vi "Autonomous Independent.vi"() -> ()   [LabVIEW 2016]
doc: "This VI is called when autonomous begins, and will automatically be terminated when autonomous ends. You can carry out timed or sensor driven robot movement independently without needing to return to the caller."
uses:
  <vilib>/Rock Robotics/WPI/Utilities/WPI_GetSetVariantRefNum.vi
  <vilib>/Rock Robotics/Network Tables/NT Read String.vi
  <vilib>/Rock Robotics/WPI/RobotDrive/WPI_RobotDriveArcadeDrive_Standard(NoSaturation).vi
  <vilib>/Rock Robotics/Network Tables/NT Write Numeric Array.vi
  <vilib>/Rock Robotics/Network Tables/NT Read Number.vi
  <vilib>/Rock Robotics/WPI/Ultrasonic/WPI_SonarMB1010AnalogRefNum Registry Get.vi
  <vilib>/Rock Robotics/WPI/Ultrasonic/WPI_SonarMB1010AnalogGetRange.vi
panel:
  out "Angle":dbl
  in  "Dial":dbl(knob) scale=-180.0..180.0
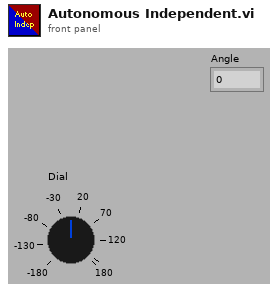
[diagram p1: front panel]
types:
  T1 = typedef "WPI_JoystickDevRef.ctl" = cluster{"Device":T2}
  T2 = typedef "WPI_JoystickDeviceEnum.ctl" = enum16{"USB 0", "USB 1", "USB 2", "USB 3", "USB 4", "USB 5"}
  T3 = typedef "WPI_RobotDriveDevRef.ctl" = cluster{"DevStatus":errorcluster, "Motors[]":T4[], "Square Inputs":bool, "Max Output":dbl}
  T4 = typedef "WPI_MotorControlDeviceRef.ctl" = cluster{"DeviceStatus":errorcluster, "Type":T5, "PWM":cluster{"PWM Channel":T6, "DeadBand":T7}, "CAN":cluster{"Device Number":u8, "SetOutput VI Ref":variant, "GetOutput VI Ref":variant, "Enable VI Ref":variant, "Disable VI Ref":variant, "Data":variant}, "Invert":bool}
  T5 = typedef "WPI_MotorControlType.ctl" = enum16{"PWM", "CAN"}
  T6 = typedef "FPGA_DIOPWMChannel.ctl" = enum8{"PWM 0", "PWM 1", "PWM 2", "PWM 3", "PWM 4", "PWM 5", "PWM 6", "PWM 7", "PWM 8", "PWM 9", "PWM MXP 0", "PWM MXP 1", "PWM MXP 2", "PWM MXP 3", "PWM MXP 4", "PWM MXP 5", "PWM MXP 6", "PWM MXP 7", "PWM MXP 8", "PWM MXP 9", "Invalid"}
  T7 = typedef "WPI_PWMDeadband.ctl" = cluster{"Name":string, "maxPositivePwm":i32, "minPositivePwm":i32, "centerPwm":i32, "maxNegativePwm":i32, "minNegativePwm":i32, "angularRange":u16}
  T8 = typedef "WPI_SonarMB1010AnalogDeviceRef.ctl" = cluster{"AIDeviceRef":T9, "Scaling factor (V/in)":dbl, "Average Bits":u8}
  T9 = typedef "WPI_AnalogChannelDevRef.ctl" = cluster{"DevStatus":errorcluster, "Analog Channel":T10}
  T10 = typedef "FPGA_AIChannel.ctl" = enum8{"AI 0", "AI 1", "AI 2", "AI 3", "AI MXP 0", "AI MXP 1", "AI MXP 2", "AI MXP 3", "Invalid"}
  T11 = typedef "WPI_GyroDevRef.ctl" = cluster{"DevStatus":errorcluster, "Analog Channel":T10, "Offset":dbl, "Gain (VoltsPerDegree/Second)":dbl, "Gyro Type":enum16{"Analog", "XRS450"}, "Handle":i32, "SPI Bus":T12, "Device Found":bool, "Sample Rate":dbl, "Calibrate On Open":bool}
  T12 = typedef "spi_bus.ctl" = enum16{"SPI On-Board, CS0", "SPI On-Board, CS1", "SPI On-Board, CS2", "SPI On-Board, CS3", "SPI MXP", "Invalid"}
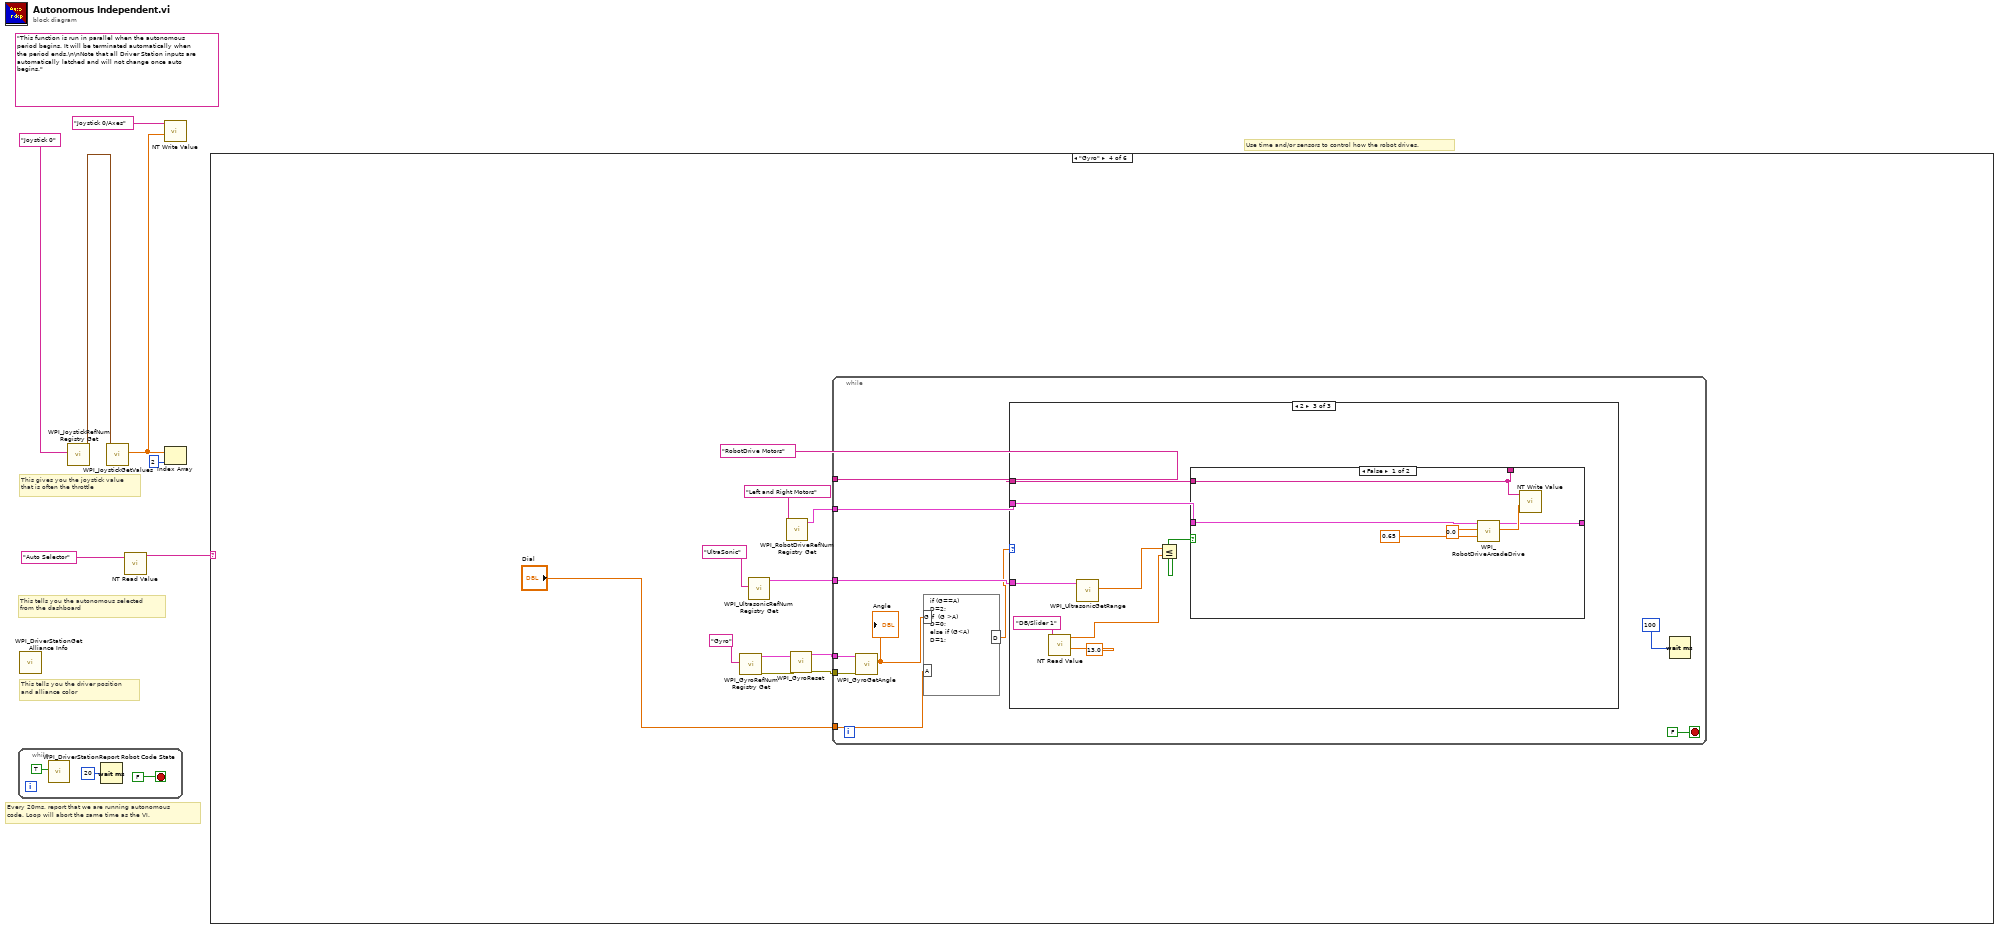
[diagram p0: block diagram]
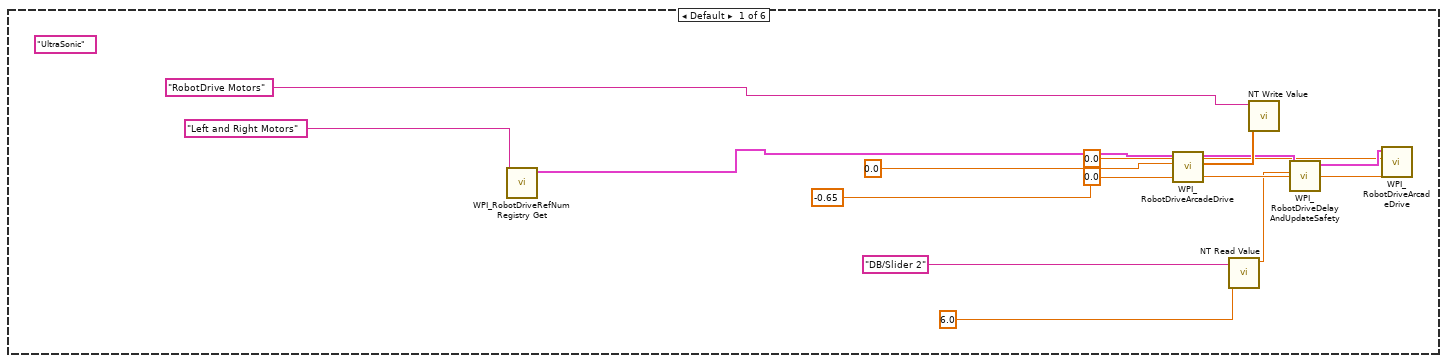
[diagram p2: hidden frame]
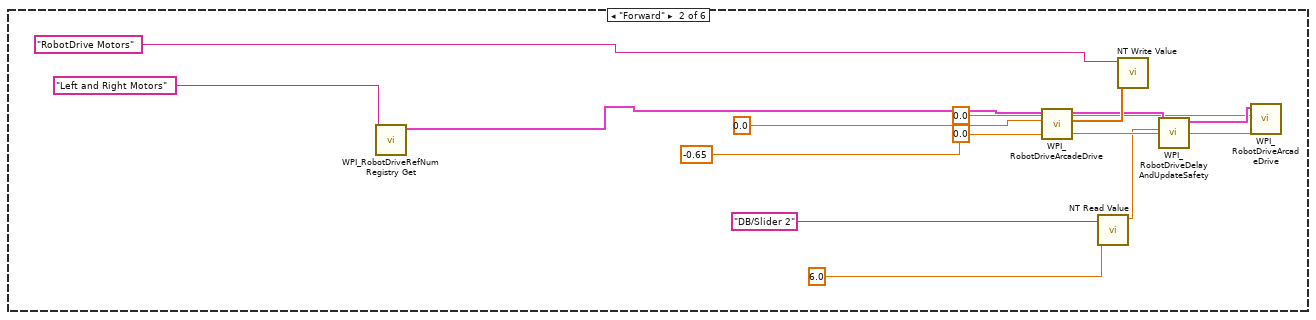
[diagram p3: hidden frame]
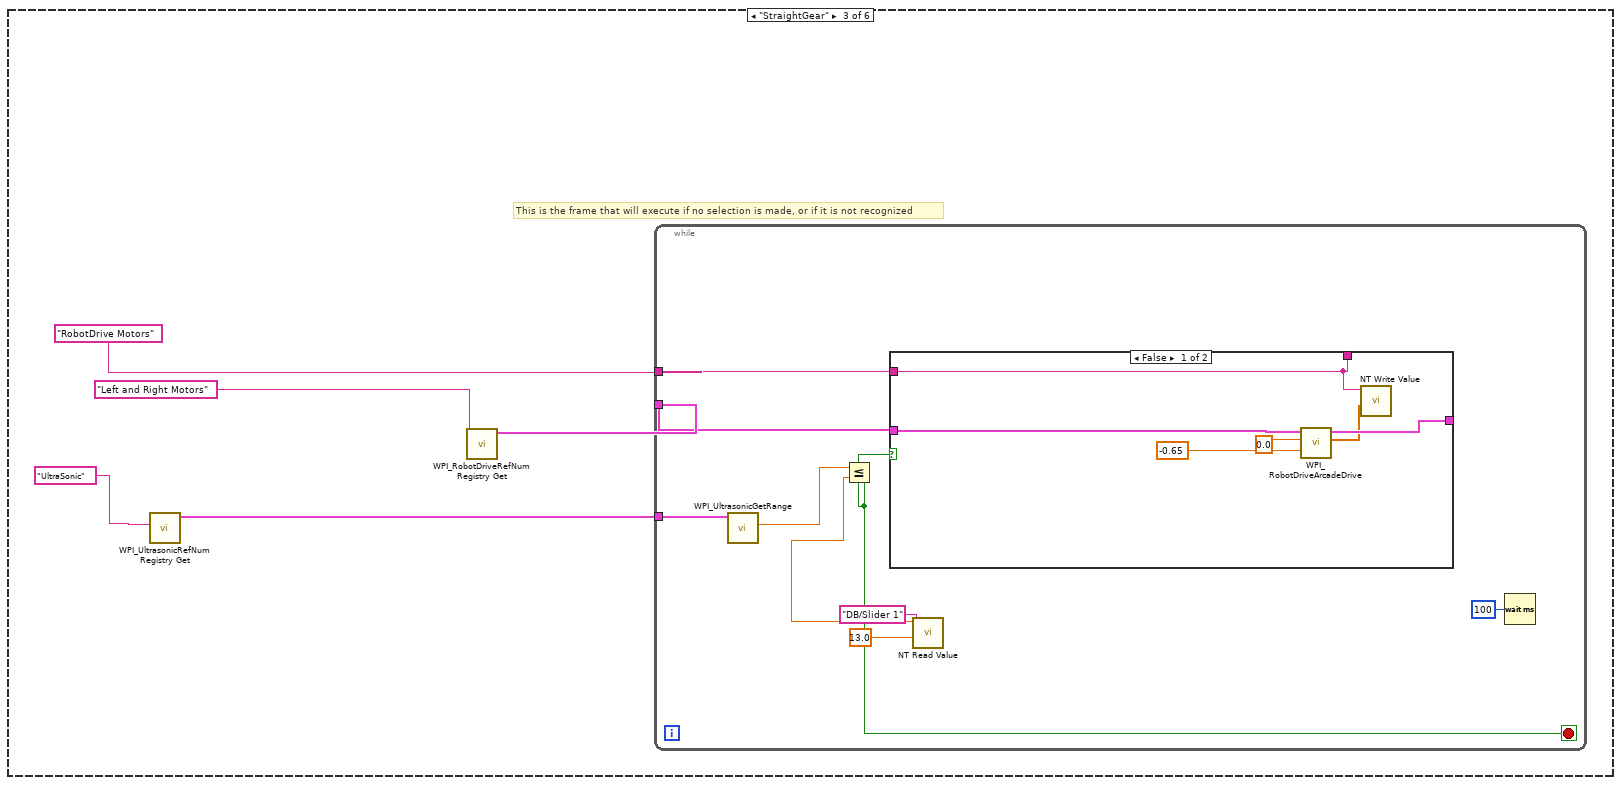
[diagram p4: hidden frame]
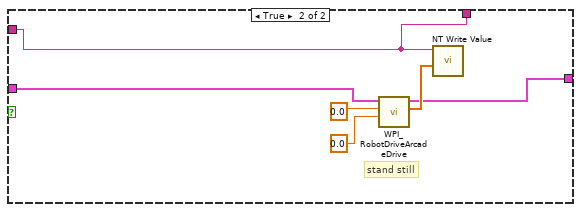
[diagram p5: hidden frame]
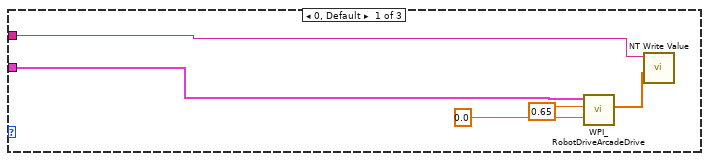
[diagram p6: hidden frame]
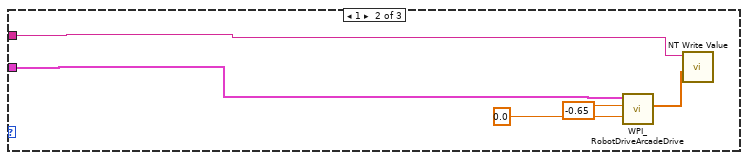
[diagram p7: hidden frame]
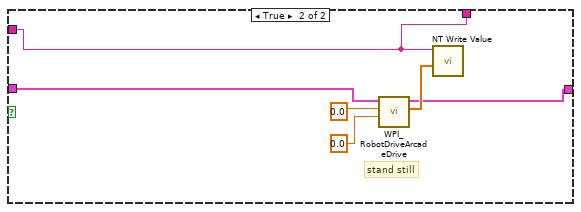
[diagram p8: hidden frame]
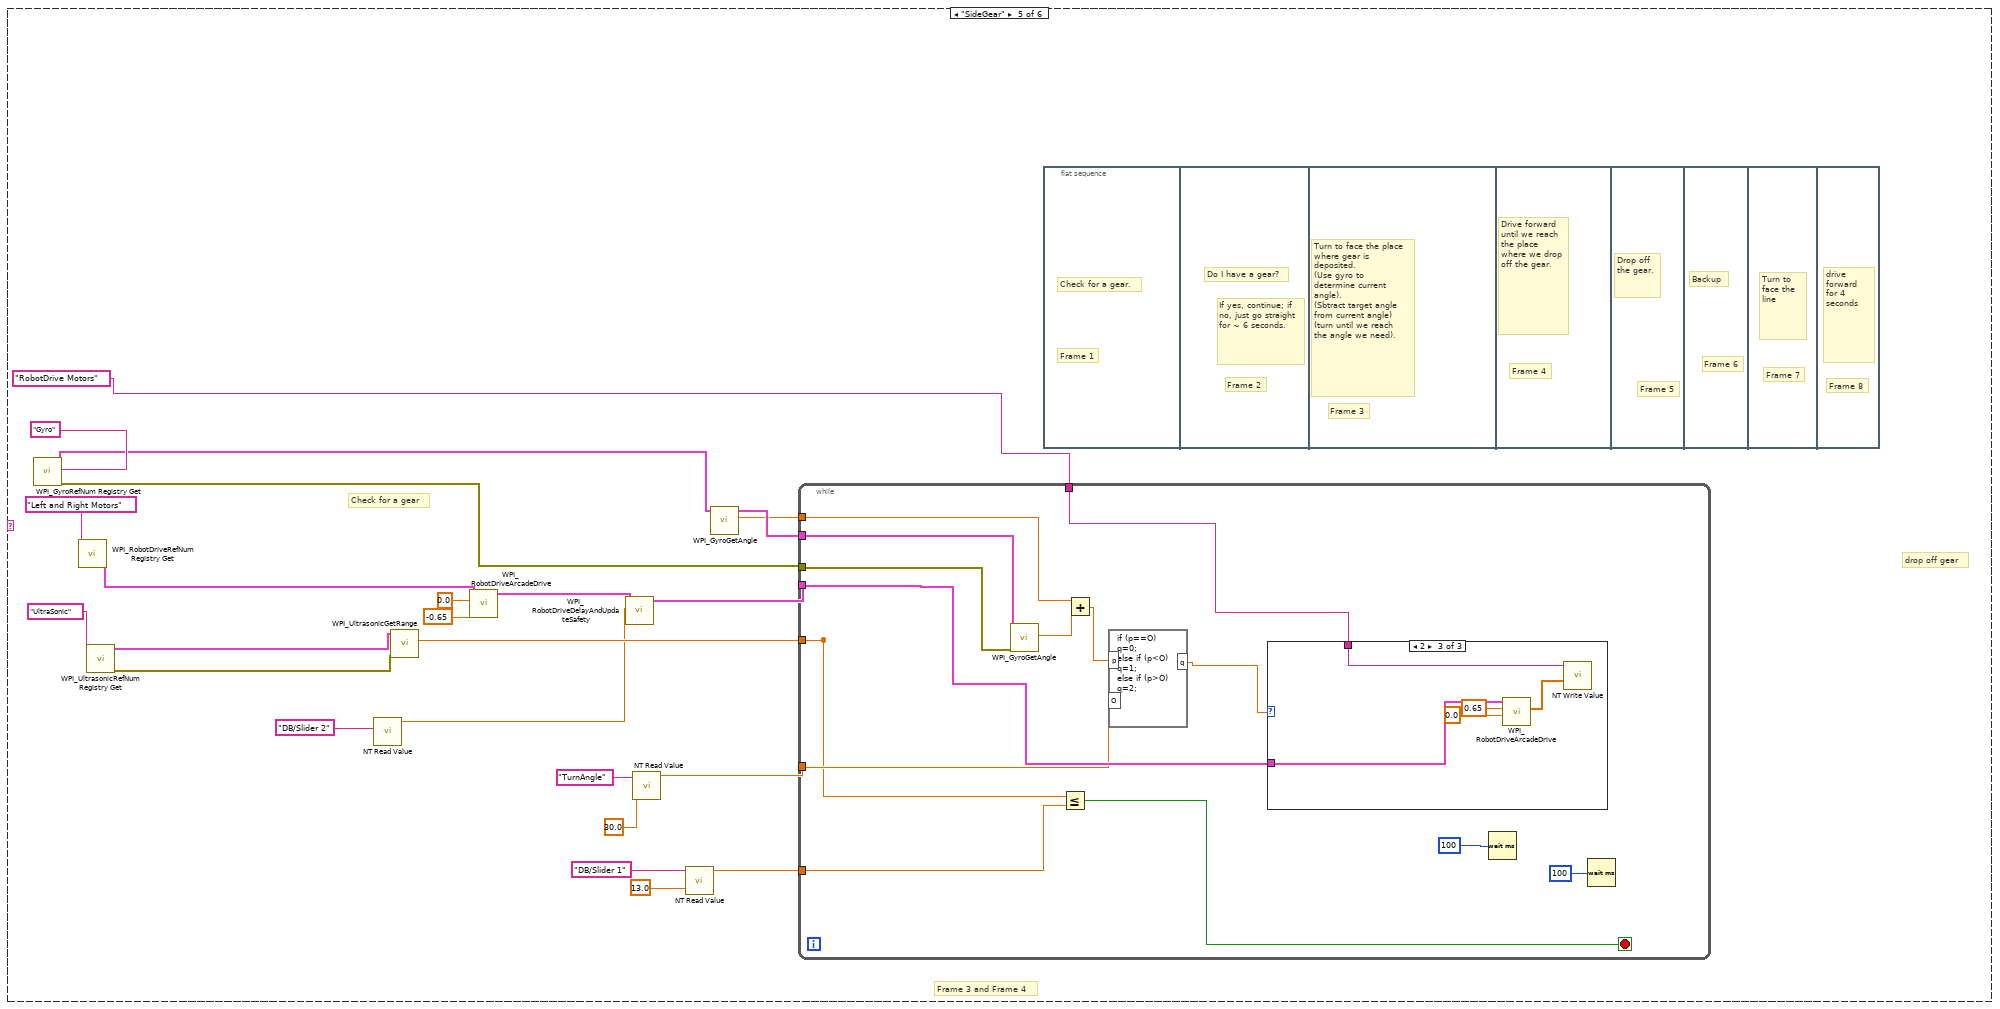
[diagram p9: hidden frame]
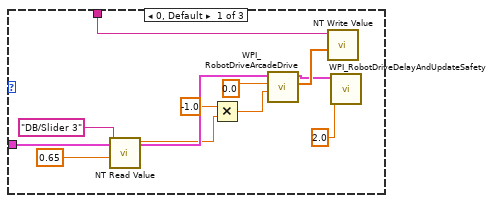
[diagram p10: hidden frame]
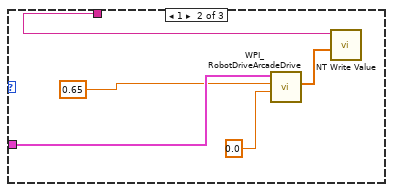
[diagram p11: hidden frame]
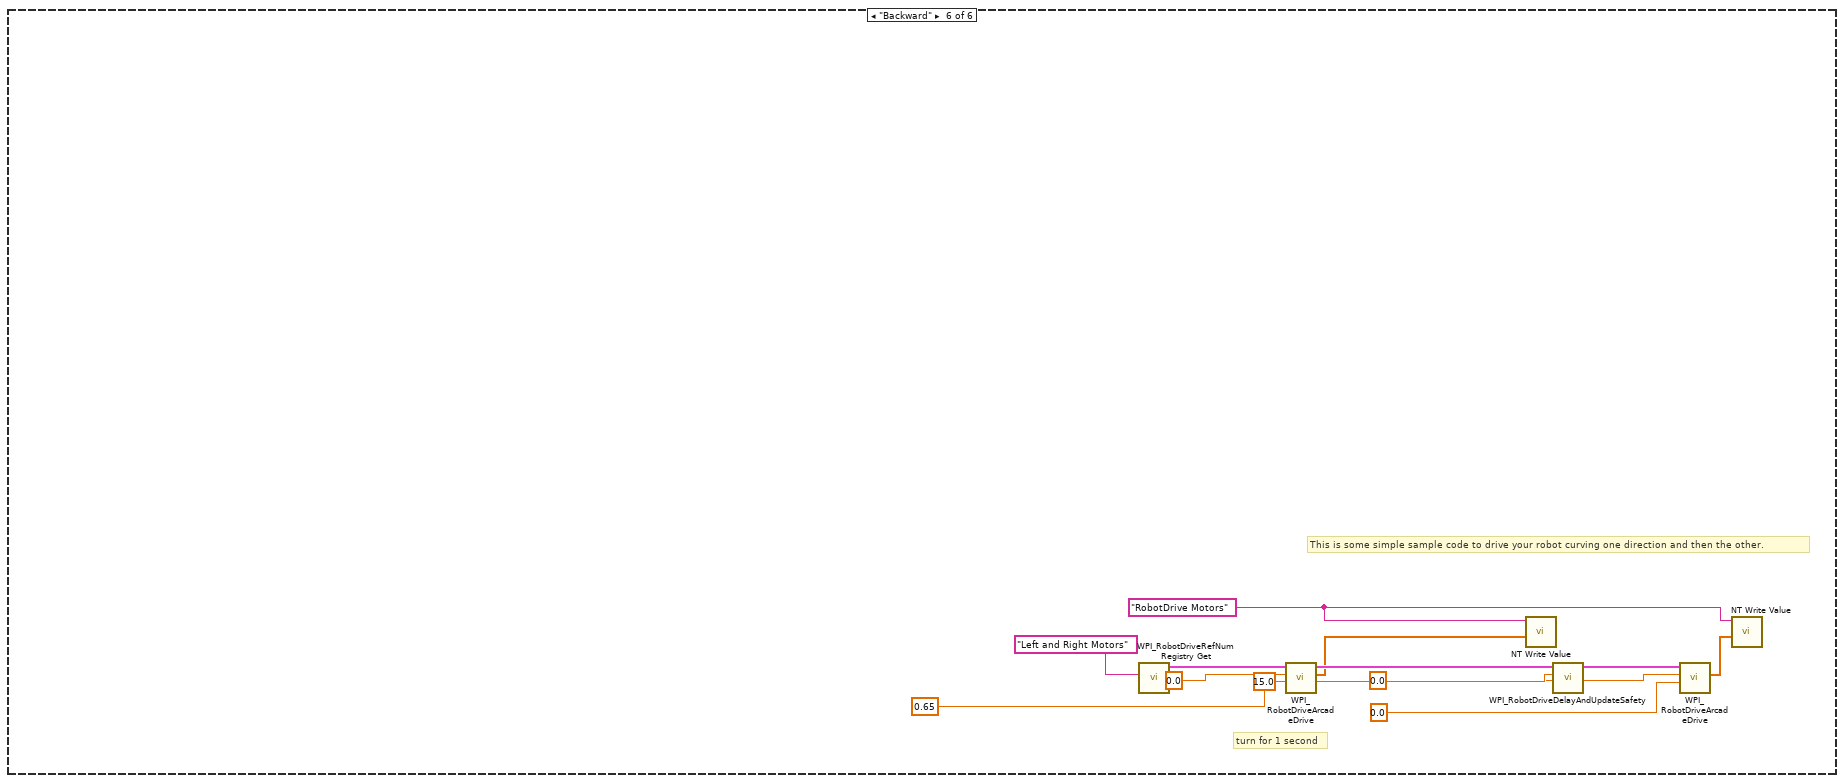
[diagram p12: hidden frame]
diagram:
  (unwired) "This function is run in parallel when the autonomous period begins. It will be terminated automatically when the period ends.\n\nNote that all Driver Station inputs are automatically latched and will not change once auto begins."
  # "This tells you the autonomous selected\nfrom the dashboard"
  # "Every 20ms, report that we are running autonomous\ncode. Loop will abort the same time as the VI."
  # "This gives you the joystick value\nthat is often the throttle"
  # "Use time and/or sensors to control how the robot drives."
  # "This tells you the driver position\nand alliance color"
  n1 = while {
    stop <- FALSE stop-if-true
    n2 = call <vilib>:"WPI_DriverStationReport Robot Code State.vi"("Autonomous"=TRUE) -> ()  [unwired: 10 in, 1 out]
    n3 = Wait (ms)(milliseconds to wait=u32 20) -> ()  [unwired: 1 out]
  }
  n4 = call <vilib>:"WPI_DriverStationGet Alliance Info.vi"() -> ()  [unwired: 12 out]
  n5 = call <vilib>:"WPI_JoystickRefNum Registry Get.vi"("refnum name"="Joystick 0") -> ("JoystickDevRef"=w6:T1)  [unwired: 1 in, 9 out]
  n6 = call <vilib>:"WPI_JoystickGetValues.vi"("JoystickDevRef"=w6) -> ("Axes"=w2:dbl[])  [unwired: 6 in, 4 out]
  n7 = call-poly <vilib>:"NT Read Value.vi"("Name"="Auto Selector") -> ("String"=w3:string)  [unwired: 9 in, 1 out]
  n8 = call-poly <vilib>:"NT Write Value.vi"("Numeric Array"=w2, "Name"="Joystick 0/Axes") -> ()  [unwired: 9 in, 1 out]
  n9 = Index Array(array=w2, index=2) -> ()  [unwired: 1 out]
  n10 = case shown="\"Gyro\"" w3 {
    frame Default {
      (unwired) "UltraSonic" ("refnum name")
      n11 = call <vilib>:"WPI_RobotDriveRefNum Registry Get.vi"("refnum name"="Left and Right Motors") -> ("RobotDriveDevRef"=w19:T3)  [unwired: 1 in, 9 out]
      n12 = call-poly <vilib>:"WPI_RobotDriveArcadeDrive.vi"("Y axis value"=-0.65, "X axis value"=0.0, "RobotDriveDevRef"=w19) -> ("Motor Values"=w20:dbl[], "RobotDriveDevRef"=w17:T3)  [unwired: 1 in, 6 out]
      n13 = call-poly <vilib>:"NT Read Value.vi"("Default Value"=6.0, "Name"="DB/Slider 2") -> ("Numeric"=w13:dbl)  [unwired: 8 in, 1 out]
      n14 = call-poly <vilib>:"NT Write Value.vi"("Numeric Array"=w20, "Name"="RobotDrive Motors") -> ()  [unwired: 9 in, 1 out]
      n15 = call <vilib>:"WPI_RobotDriveDelayAndUpdateSafety.vi"("Delay (s)"=w13, "RobotDriveDevRef"=w17) -> ("RobotDriveDevRef 2"=w16:T3)  [unwired: 8 in, 1 out]
      n16 = call-poly <vilib>:"WPI_RobotDriveArcadeDrive.vi"("Y axis value"=0.0, "X axis value"=0.0, "RobotDriveDevRef"=w16) -> ()  [unwired: 1 in, 8 out]
    }
    frame "Forward" {
      n17 = call <vilib>:"WPI_RobotDriveRefNum Registry Get.vi"("refnum name"="Left and Right Motors") -> ("RobotDriveDevRef"=w32:T3)  [unwired: 1 in, 9 out]
      n18 = call-poly <vilib>:"WPI_RobotDriveArcadeDrive.vi"("Y axis value"=-0.65, "X axis value"=0.0, "RobotDriveDevRef"=w32) -> ("Motor Values"=w33:dbl[], "RobotDriveDevRef"=w30:T3)  [unwired: 1 in, 6 out]
      n19 = call-poly <vilib>:"NT Read Value.vi"("Default Value"=6.0, "Name"="DB/Slider 2") -> ("Numeric"=w26:dbl)  [unwired: 8 in, 1 out]
      n20 = call-poly <vilib>:"NT Write Value.vi"("Numeric Array"=w33, "Name"="RobotDrive Motors") -> ()  [unwired: 9 in, 1 out]
      n21 = call <vilib>:"WPI_RobotDriveDelayAndUpdateSafety.vi"("Delay (s)"=w26, "RobotDriveDevRef"=w30) -> ("RobotDriveDevRef 2"=w29:T3)  [unwired: 8 in, 1 out]
      n22 = call-poly <vilib>:"WPI_RobotDriveArcadeDrive.vi"("Y axis value"=0.0, "X axis value"=0.0, "RobotDriveDevRef"=w29) -> ()  [unwired: 1 in, 8 out]
    }
    frame "StraightGear" {
      # "This is the frame that will execute if no selection is made, or if it is not recognized"
      n23 = call-poly <vilib>:"WPI_UltrasonicRefNum Registry Get.vi"("refnum name"="UltraSonic") -> ("SonarMB1010AnalogDevRef"=w38:T8)  [unwired: 9 in, 1 out]
      n24 = call <vilib>:"WPI_RobotDriveRefNum Registry Get.vi"("refnum name"="Left and Right Motors") -> ("RobotDriveDevRef"=w39:T3)  [unwired: 1 in, 9 out]
      n25 = while {
        tunnel: "RobotDrive Motors" ("Name") -> [w50]
        tunnel: w39 -> [w49]
        tunnel: w38 -> [w47]
        stop <- w42 stop-if-true
        n26 = call-poly <vilib>:"WPI_UltrasonicGetRange.vi"("SonarMB1010AnalogDevRef"=w47) -> ("Distance"=w48:dbl)  [unwired: 8 in, 2 out]
        n27 = call-poly <vilib>:"NT Read Value.vi"("Default Value"=13.0, "Name"="DB/Slider 1") -> ("Numeric"=w43:dbl)  [unwired: 8 in, 1 out]
        n28 = Less Or Equal?(x=w48, y=w43) -> (x <= y?=w42:bool)
        n29 = case shown="False" w42 {
          tunnel: w50 -> [w55 w57]
          tunnel: [w55 w57] -> _
          tunnel: w49 -> [w54 w59]
          tunnel: [w53 w58] -> _
          frame False {
            n30 = call-poly <vilib>:"WPI_RobotDriveArcadeDrive.vi"("Y axis value"=-0.65, "X axis value"=0.0, "RobotDriveDevRef"=w54) -> ("Motor Values"=w51:dbl[], "RobotDriveDevRef"=w53:T3)  [unwired: 1 in, 6 out]
            n31 = call-poly <vilib>:"NT Write Value.vi"("Numeric Array"=w51, "Name"=w55) -> ()  [unwired: 9 in, 1 out]
          }
          frame True {
            # "stand still"
            n32 = call-poly <vilib>:"WPI_RobotDriveArcadeDrive.vi"("Y axis value"=0.0 ("X axis value"), "X axis value"=0.0, "RobotDriveDevRef"=w59) -> ("Motor Values"=w62:dbl[], "RobotDriveDevRef"=w58:T3)  [unwired: 1 in, 6 out]
            n33 = call-poly <vilib>:"NT Write Value.vi"("Numeric Array"=w62, "Name"=w57) -> ()  [unwired: 9 in, 1 out]
          }
        }
        n34 = Wait (ms)(milliseconds to wait=u32 100) -> ()  [unwired: 1 out]
      }
    }
    frame "Gyro" {
      n35 = call <vilib>:"WPI_GyroRefNum Registry Get.vi"("refnum name"="Gyro") -> ("error out"=w66:errorcluster, "GyroDevRef"=w65:T11)  [unwired: 9 in]
      n36 = call-poly <vilib>:"WPI_UltrasonicRefNum Registry Get.vi"("refnum name"="UltraSonic") -> ("SonarMB1010AnalogDevRef"=w71:T8)  [unwired: 9 in, 1 out]
      n37 = call <vilib>:"WPI_RobotDriveRefNum Registry Get.vi"("refnum name"="Left and Right Motors") -> ("RobotDriveDevRef"=w68:T3)  [unwired: 1 in, 9 out]
      n38 = call <vilib>:"WPI_GyroReset.vi"("error in"=w66, "GyroDevRef"=w65) -> ("error out"=w67:errorcluster, "GyroDevRef"=w64:T11)  [unwired: 8 in]
      n39 = while {
        tunnel: "RobotDrive Motors" ("Name") -> [w83]
        tunnel: w68 -> [w79]
        tunnel: w71 -> [w77]
        tunnel: w64 -> [w81]
        tunnel: w67 -> [w80]
        tunnel: "Dial" -> [w75]
        stop <- FALSE stop-if-true
        n40 = call <vilib>:"WPI_GyroGetAngle.vi"("error in"=w80, "GyroDevRef"=w81) -> ("Angle"=w74:dbl)  [unwired: 5 in, 4 out]
        "Angle" <- w74
        n41 = formula code="if (G==A)\nD=2;\nif  (G >A)\nD=0;\nelse if (G<A)\nD=1;"("G"=w74, "A"=w75) -> ("D"=w76:dbl)
        n42 = case shown="2" w76 {
          tunnel: w83 -> [w84 w90 w100]
          tunnel: w79 -> [w85 w89 w99]
          tunnel: w77 -> [_ _ w97]
          frame 0, Default {
            n43 = call-poly <vilib>:"WPI_RobotDriveArcadeDrive.vi"("Y axis value"=0.0, "X axis value"=0.65, "RobotDriveDevRef"=w85) -> ("Motor Values"=w88:dbl[])  [unwired: 1 in, 7 out]
            n44 = call-poly <vilib>:"NT Write Value.vi"("Numeric Array"=w88, "Name"=w84) -> ()  [unwired: 9 in, 1 out]
          }
          frame 1 {
            n45 = call-poly <vilib>:"WPI_RobotDriveArcadeDrive.vi"("Y axis value"=0.0, "X axis value"=-0.65, "RobotDriveDevRef"=w89) -> ("Motor Values"=w91:dbl[])  [unwired: 1 in, 7 out]
            n46 = call-poly <vilib>:"NT Write Value.vi"("Numeric Array"=w91, "Name"=w90) -> ()  [unwired: 9 in, 1 out]
          }
          frame 2 {
            n47 = call-poly <vilib>:"NT Read Value.vi"("Default Value"=13.0, "Name"="DB/Slider 1") -> ("Numeric"=w94:dbl)  [unwired: 8 in, 1 out]
            n48 = call-poly <vilib>:"WPI_UltrasonicGetRange.vi"("SonarMB1010AnalogDevRef"=w97) -> ("Distance"=w98:dbl)  [unwired: 8 in, 2 out]
            n49 = Less Or Equal?(x=w98, y=w94) -> (x <= y?=w101:bool)
            n50 = case shown="False" w101 {
              tunnel: w100 -> [w106 w109]
              tunnel: [w106 w109] -> _
              tunnel: w99 -> [w105 w110]
              tunnel: [w102 w108] -> _
              frame False {
                n51 = call-poly <vilib>:"WPI_RobotDriveArcadeDrive.vi"("Y axis value"=0.65, "X axis value"=0.0, "RobotDriveDevRef"=w105) -> ("Motor Values"=w103:dbl[], "RobotDriveDevRef"=w102:T3)  [unwired: 1 in, 6 out]
                n52 = call-poly <vilib>:"NT Write Value.vi"("Numeric Array"=w103, "Name"=w106) -> ()  [unwired: 9 in, 1 out]
              }
              frame True {
                # "stand still"
                n53 = call-poly <vilib>:"WPI_RobotDriveArcadeDrive.vi"("Y axis value"=0.0 ("X axis value"), "X axis value"=0.0, "RobotDriveDevRef"=w110) -> ("Motor Values"=w113:dbl[], "RobotDriveDevRef"=w108:T3)  [unwired: 1 in, 6 out]
                n54 = call-poly <vilib>:"NT Write Value.vi"("Numeric Array"=w113, "Name"=w109) -> ()  [unwired: 9 in, 1 out]
              }
            }
          }
        }
        n55 = Wait (ms)(milliseconds to wait=u32 100) -> ()  [unwired: 1 out]
      }
    }
    frame "SideGear" {
      # "Check for a gear"
      # "Frame 3 and Frame 4"
      # "drop off gear"
      n56 = call <vilib>:"WPI_GyroRefNum Registry Get.vi"("refnum name"="Gyro") -> ("error out"=w132:errorcluster, "GyroDevRef"=w122:T11)  [unwired: 9 in]
      n57 = call <vilib>:"WPI_RobotDriveRefNum Registry Get.vi"("refnum name"="Left and Right Motors") -> ("RobotDriveDevRef"=w129:T3)  [unwired: 1 in, 9 out]
      n58 = call-poly <vilib>:"WPI_UltrasonicRefNum Registry Get.vi"("refnum name"="UltraSonic") -> ("error out"=w130:errorcluster, "SonarMB1010AnalogDevRef"=w134:T8)  [unwired: 9 in]
      n59 = call-poly <vilib>:"NT Read Value.vi"("Name"="DB/Slider 2") -> ("Numeric"=w124:dbl)  [unwired: 9 in, 1 out]
      n60 = call-poly <vilib>:"WPI_UltrasonicGetRange.vi"("error in"=w130, "SonarMB1010AnalogDevRef"=w134) -> ("Distance"=w133:dbl)  [unwired: 7 in, 2 out]
      n61 = call-poly <vilib>:"WPI_RobotDriveArcadeDrive.vi"("Y axis value"=-0.65, "X axis value"=0.0, "RobotDriveDevRef"=w129) -> ("RobotDriveDevRef"=w126:T3)  [unwired: 6 in, 2 out]
      n62 = call <vilib>:"WPI_RobotDriveDelayAndUpdateSafety.vi"("Delay (s)"=w124, "RobotDriveDevRef"=w126) -> ("RobotDriveDevRef 2"=w127:T3)  [unwired: 8 in, 1 out]
      n63 = call-poly <vilib>:"NT Read Value.vi"("Default Value"=30.0, "Name"="TurnAngle") -> ("Numeric"=w118:dbl)  [unwired: 8 in, 1 out]
      n64 = call-poly <vilib>:"NT Read Value.vi"("Default Value"=13.0, "Name"="DB/Slider 1") -> ("Numeric"=w116:dbl)  [unwired: 8 in, 1 out]
      n65 = call <vilib>:"WPI_GyroGetAngle.vi"("GyroDevRef"=w122) -> ("Angle"=w120:dbl, "GyroDevRef"=w121:T11)  [unwired: 6 in, 3 out]
      n66 = while {
        tunnel: w121 -> [w150]
        tunnel: w127 -> [w149]
        tunnel: "RobotDrive Motors" ("Name") -> [w145]
        tunnel: w132 -> [w148]
        tunnel: [w143] -> _
        tunnel: w118 -> [w144]
        tunnel: w133 -> [w143]
        tunnel: w120 -> [w142]
        tunnel: w116 -> [w139]
        stop <- w146 stop-if-true
        n67 = call <vilib>:"WPI_GyroGetAngle.vi"("error in"=w148, "GyroDevRef"=w150) -> ("Angle"=w141:dbl)  [unwired: 5 in, 4 out]
        n68 = Less Or Equal?(x=w143, y=w139) -> (x <= y?=w146:bool)
        n69 = Add(x=w142, y=w141) -> (x+y=w140:dbl)
        n70 = formula code="if (p==O)\nq=0;\nelse if (p<O)\nq=1;\nelse if (p>O)\nq=2;"("p"=w140, "O"=w144) -> ("q"=w147:dbl)
        n71 = case shown="2" w147 {
          tunnel: w149 -> [w158 w166 w171]
          tunnel: w145 -> [w157 w165 w168]
          frame 0, Default {
            n72 = call-poly <vilib>:"NT Read Value.vi"("Default Value"=0.65, "Name"="DB/Slider 3") -> ("Numeric"=w155:dbl)  [unwired: 8 in, 1 out]
            n73 = Multiply(x=-1.0, y=w155) -> (x*y=w156:dbl)
            n74 = call-poly <vilib>:"WPI_RobotDriveArcadeDrive.vi"("Y axis value"=w156, "X axis value"=0.0, "RobotDriveDevRef"=w158) -> ("Motor Values"=w160:dbl[], "RobotDriveDevRef"=w152:T3)  [unwired: 1 in, 6 out]
            n75 = call-poly <vilib>:"NT Write Value.vi"("Numeric Array"=w160, "Name"=w157) -> ()  [unwired: 9 in, 1 out]
            n76 = call <vilib>:"WPI_RobotDriveDelayAndUpdateSafety.vi"("Delay (s)"=2.0, "RobotDriveDevRef"=w152) -> ()  [unwired: 8 in, 2 out]
          }
          frame 1 {
            n77 = call-poly <vilib>:"WPI_RobotDriveArcadeDrive.vi"("Y axis value"=0.0, "X axis value"=0.65 ("Default Value"), "RobotDriveDevRef"=w166) -> ("Motor Values"=w167:dbl[])  [unwired: 1 in, 7 out]
            n78 = call-poly <vilib>:"NT Write Value.vi"("Numeric Array"=w167, "Name"=w165) -> ()  [unwired: 9 in, 1 out]
          }
          frame 2 {
            n79 = call-poly <vilib>:"WPI_RobotDriveArcadeDrive.vi"("Y axis value"=0.0, "X axis value"=0.65, "RobotDriveDevRef"=w171) -> ("Motor Values"=w172:dbl[])  [unwired: 1 in, 7 out]
            n80 = call-poly <vilib>:"NT Write Value.vi"("Numeric Array"=w172, "Name"=w168) -> ()  [unwired: 9 in, 1 out]
          }
        }
        n81 = Wait (ms)(milliseconds to wait=u32 100) -> ()  [unwired: 1 out]
      }
      n82 = flat-sequence {
        frame #0 {
          # "Frame 1"
          # "Check for a gear."
        }
        frame #1 {
          # "Frame 2"
          # "If yes, continue; if no, just go straight for ~ 6 seconds."
          # "Do I have a gear?"
        }
        frame #2 {
          # "Frame 3"
          # "Turn to face the place where gear is deposited.\n(Use gyro to determine current angle).\n(Sbtract target angle from current angle)\n(turn until we reach the angle we need)."
        }
        frame #3 {
          # "Drive forward until we reach the place where we drop off the gear."
          # "Frame 4"
        }
        frame #4 {
          # "Frame 5"
          # "Drop off the gear."
        }
        frame #5 {
          # "Frame 6"
          # "Backup"
        }
        frame #6 {
          # "Frame 7"
          # "Turn to face the line"
        }
        frame #7 {
          # "Frame 8"
          # "drive forward for 4 seconds"
        }
      }
      n83 = Wait (ms)(milliseconds to wait=u32 100) -> ()  [unwired: 1 out]
    }
    frame "Backward" {
      w175 = "RobotDrive Motors" ("Name")
      # "This is some simple sample code to drive your robot curving one direction and then the other."
      # "turn for 1 second"
      n84 = call <vilib>:"WPI_RobotDriveRefNum Registry Get.vi"("refnum name"="Left and Right Motors") -> ("RobotDriveDevRef"=w184:T3)  [unwired: 1 in, 9 out]
      n85 = call-poly <vilib>:"WPI_RobotDriveArcadeDrive.vi"("Y axis value"=0.65 ("Default Value"), "X axis value"=0.0, "RobotDriveDevRef"=w184) -> ("Motor Values"=w174:dbl[], "RobotDriveDevRef"=w180:T3)  [unwired: 1 in, 6 out]
      n86 = call-poly <vilib>:"NT Write Value.vi"("Numeric Array"=w174, "Name"=w175) -> ()  [unwired: 9 in, 1 out]
      n87 = call <vilib>:"WPI_RobotDriveDelayAndUpdateSafety.vi"("Delay (s)"=15.0, "RobotDriveDevRef"=w180) -> ("RobotDriveDevRef 2"=w181:T3)  [unwired: 8 in, 1 out]
      n88 = call-poly <vilib>:"WPI_RobotDriveArcadeDrive.vi"("Y axis value"=0.0 ("X axis value"), "X axis value"=0.0, "RobotDriveDevRef"=w181) -> ("Motor Values"=w176:dbl[])  [unwired: 1 in, 7 out]
      n89 = call-poly <vilib>:"NT Write Value.vi"("Numeric Array"=w176, "Name"=w175) -> ()  [unwired: 9 in, 1 out]
    }
  }
